vi "Blackman-Nuttall Window (DBL).vi"(11 "X":dbl[](array[numeric])) -> (0 "error":i32, 3 "Windowed X":dbl[](array[numeric]))   [LabVIEW 2014, in "NI_AALPro.lvlib"]
doc: "Applies a Blackman-Nuttall window to the input sequence <B>X</B>. Wire data to the <B>X</B> input to determine the polymorphic instance to use or manually select the instance."
uses:
  NI_AALPro.lvlib
panel:
  # "Blackman-Nuttall Window"
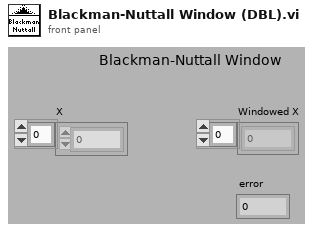
[diagram p1: front panel]
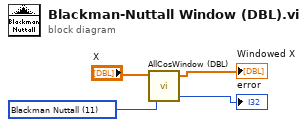
[diagram p0: block diagram]
diagram:
  w1 = u16 11 items=["None "=0, "Hanning"=1, "Hamming"=2, "Blackman-Harris"=3, "Exact Blackman"=4, "Blackman"=5, "Flat Top"=6, "4 Term B-Harris "=7, "7 Term B-Harris"=8, "Low Sidelobe"=9, "Blackman Nuttall"=11] ("window")
  n1 = call "AllCosWindow (DBL).vi"("window"=w1, "X"="X") -> ("error"=→"error":i32, "Windowed X"=→"Windowed X":dbl[])  [unwired: 3 in]
